vi "TPNT_AddDeviceTP.vi"(8 "error in (no error)":errorcluster, 10 "arguments":string, 11 "Object Refnum In":T5) -> (0 "error out":errorcluster, 3 "Data Refnum out":T5)   [LabVIEW 2016]
uses:
  TPNT_Refnum.ctl
  TPNT_TP.ctl
  TPNT_Limits.ctl
  TPNT_Samples.ctl
  TPNT_Log.ctl
panel:
  in  "TP":T1={"name"="", "type"="", "algor"=[], "update_rate"=0.0, "Limits"={"Alarm Type"="", "Lower "=0.0, "Upper"=0.0, "Nominal"=0.0, "outrange"=FALSE, "Check"=TRUE, "latch"=FALSE, "level"=""}, "Samples"={"samples"=0, "counter"=0, "Values"=[], "Current Value"="", "filter"="", "precision"=2}, "next_update"=0, "Status"="", "monitor"=TRUE, "error"=FALSE, "Log"={"log"=FALSE, "file"=path "", "type"="text", "format"="name= value", "updaterate"=0.0, "nex_update"=0, "mode"=""}, "permissions"="", "ID"=""} {"Log"."updaterate" format="%.2f"; "Samples"."Values" format="%.2f"; "Samples"."samples" min=1 step=1; "Limits"."Nominal" format="%.2f"; "Limits"."Upper" format="%.2f"; "Limits"."Lower" format="%.2f"; "update_rate" format="%.2f"}
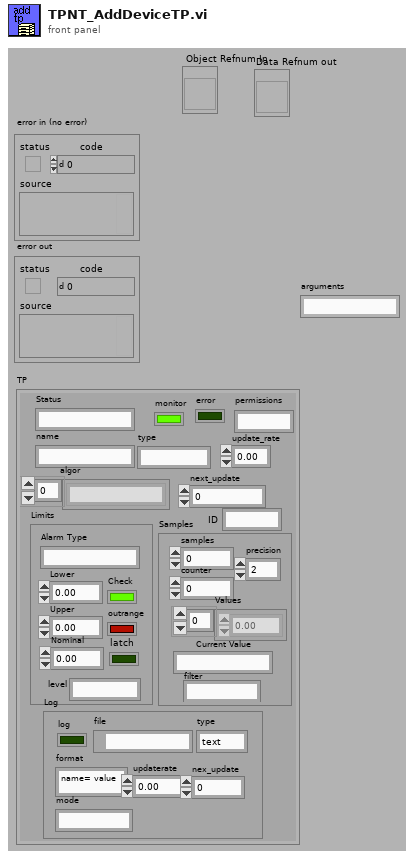
[diagram p1: front panel]
types:
  T1 = typedef "TPNT_TP.ctl" = cluster{"name":string, "type":string, "algor":string[], "update_rate":sgl, "Limits":T2, "Samples":T3, "next_update":u32, "Status":string, "monitor":bool, "error":bool, "Log":T4, "permissions":string, "ID":string}
  T2 = typedef "TPNT_Limits.ctl" = cluster{"Alarm Type":string, "Lower ":dbl, "Upper":dbl, "Nominal":dbl, "outrange":bool, "Check":bool, "latch":bool, "level":string}
  T3 = typedef "TPNT_Samples.ctl" = cluster{"samples":i32, "counter":i32, "Values":dbl[], "Current Value":string, "filter":string, "precision":u8}
  T4 = typedef "TPNT_Log.ctl" = cluster{"log":bool, "file":path, "type":string, "format":string, "updaterate":dbl, "nex_update":u32, "mode":string}
  T5 = typedef "TPNT_Refnum.ctl" = refnum<vi>
  T6 = typedef "TPNT_DeviceTPs.ctl" = cluster{"device":string, "devupdate":dbl, "next_update":u32, "devinterface":string, "TPs":T1[], "Alarms":bool, "monitor":bool, "log sep":string}
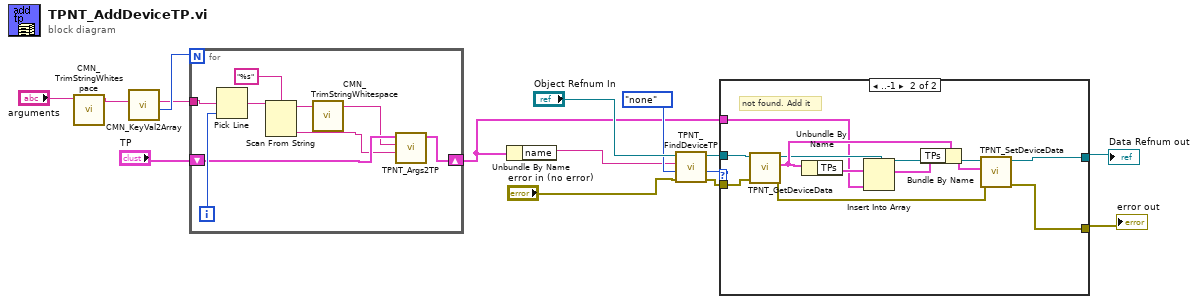
[diagram p0: block diagram]
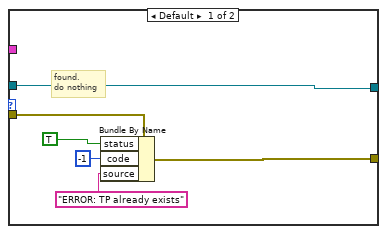
[diagram p2: hidden frame]
diagram:
  n1 = call "CMN_TrimStringWhitespace.vi"("string"="arguments") -> ("trimmed string"=w2:string)  [unwired: 1 in, 8 out]
  n2 = call "CMN_KeyVal2Array.vi"("command in"=w2) -> ("number of commands"=w6:i32, "commands out"=w5:string)  [unwired: 2 in, 6 out]
  n3 = for {
    N: w6 -> [_]
    tunnel: w5 -> [w24]
    shift-right: [w18] -> w1
    shift-left: "TP" -> [w19]
    i -> [w23]
    n4 = Pick Line(multi-line string=w24, line index=w23) -> (output string=w22:string)  [unwired: 1 out]
    n5 = Scan From String(format string="%s", input string=w22) -> (remaining string=w20:string, output 1=w16:string)  [unwired: 2 in, 3 out]
    n6 = call "CMN_TrimStringWhitespace.vi"("string"=w20) -> ("trimmed string"=w17:string)  [unwired: 1 in, 8 out]
    n7 = call "TPNT_Args2TP.vi"("key"=w16, "value"=w17, "TP_IN"=w19) -> ("TP_OUT"=w18:T1)  [unwired: 8 out]
  }
  n8 = Unbundle By Name(w1) -> ("name"=w4:string)
  n9 = call "TPNT_FindDeviceTP.vi"("error in (no error)"="error in (no error)", "error"=enum16{"none", "on found", "on not found"}."none", "TP name"=w4, "Object Refnum In"="Object Refnum In") -> ("error out"=w12:errorcluster, "index"=w15:i32, "Data Refnum out"=w10:T5)  [unwired: 5 out]
  n10 = case shown="..-1" w15 {
    tunnel: w12 -> [w29 w40]
    tunnel: [w26 w33] -> w11
    tunnel: w10 -> [w25 w41]
    tunnel: [w25 w32] -> w9
    tunnel: w1 -> [_ w31]
    frame Default {
      # "found.\ndo nothing"
      n11 = Bundle By Name(cluster=w29, "status"=TRUE, "code"=-1, "source"="ERROR: TP already exists") -> (w26:errorcluster)
    }
    frame ..-1 {
      # "not found. Add it"
      n12 = call "TPNT_GetDeviceData.vi"("error in (no error)"=w40, "Object Refnum In"=w41) -> ("error out"=w34:errorcluster, "Object Data Out"=w37:T6, "Data Refnum out"=w36:T5)  [unwired: 7 out]
      n13 = Unbundle By Name(w37) -> ("TPs"=w39:T1[])
      n14 = Insert Into Array(array=w39, new element=w31) -> (w38:T1[])  [unwired: 1 in]
      n15 = Bundle By Name(cluster=w37, "TPs"=w38) -> (w35:T6)
      n16 = call "TPNT_SetDeviceData.vi"("error in (no error)"=w34, "Object Data In"=w35, "Object Refnum In"=w36) -> ("error out"=w33:errorcluster, "Data Refnum out"=w32:T5)  [unwired: 7 out]
    }
  }
  "Data Refnum out" <- w9
  "error out" <- w11
